vi "Actor Core.vi"(8 "error in":errorcluster, 11 "Panel Object Actions UI in":refnum<class "Panel Object Actions UI.lvclass">) -> (0 "error out":errorcluster, 3 "Actor out":refnum<class "Actor.lvclass">)   [LabVIEW 2015, in "Panel Object Actions UI.lvlib" / "Panel Object Actions UI.lvclass"]
doc: "The user interface for this panel.\n\n----\nPlease see the following web address for additional documentation and tutorial information:\nhttp://www.mooregoodideas.com/mgi-panel-manager/\n\nAuthor: Derek Trepanier\n\nCopyright (c) 2018, Moore Good Ideas, Inc.\n\nAll rights reserved.\n\nRedistribution and use in source and binary forms, with or without modification, are permitted provided that the following conditions are met:\n\n * Redistributions of source code must retain the above copyright notice, this list of conditions and the following disclaimer.\n * Redistributions in binary form must reproduce the above copyright notice, this list of conditions and the following disclaimer in the documentation and/or other materials provided with the distribution.\n * Neither the name of Moore Good Ideas, Inc. nor the names of its contributors may be used to endorse or promote products derived from this software without specific prior written permission.\n\nTHIS SOFTWARE IS PROVIDED BY THE COPYRIGHT HOLDERS AND CONTRIBUTORS \"AS IS\" AND ANY EXPRESS OR IMPLIED WARRANTIES, INCLUDING, BUT NOT LIMITED TO, THE IMPLIED WARRANTIES OF MERCHANTABILITY AND FITNESS FOR A PARTICULAR PURPOSE ARE DISCLAIMED. IN NO EVENT SHALL THE COPYRIGHT OWNER OR CONTRIBUTORS BE LIABLE FOR ANY DIRECT, INDIRECT, INCIDENTAL, SPECIAL, EXEMPLARY, OR CONSEQUENTIAL DAMAGES (INCLUDING, BUT NOT LIMITED TO, PROCUREMENT OF SUBSTITUTE GOODS OR SERVICES; LOSS OF USE, DATA, OR PROFITS; OR BUSINESS INTERRUPTION) HOWEVER CAUSED AND ON ANY THEORY OF LIABILITY, WHETHER IN CONTRACT, STRICT LIABILITY, OR TORT (INCLUDING NEGLIGENCE OR OTHERWISE) ARISING IN ANY WAY OUT OF THE USE OF THIS SOFTWARE, EVEN IF ADVISED OF THE POSSIBILITY OF SUCH DAMAGE."
uses:
  Panel Object Actions UI.lvclass
  <vilib>/ActorFramework/Actor/Actor.lvclass
  Classes/Panel Object/Panel Object.lvclass
  <vilib>/ActorFramework/Actor/Actor.lvclass/Actor.ctl
  Panel Object Actions UI.lvclass/Panel Object Actions UI.ctl
  <vilib>/ActorFramework/Message Enqueuer/Message Enqueuer.lvclass/Message Enqueuer.ctl
  Typedefs/Scrollbar Visibility--Enum.ctl
  Classes/Panel Object/Align Type--Enum.ctl
  Classes/Panel Object/Distribution Type--Enum.ctl
  <vilib>/ActorFramework/Message Enqueuer/Enqueue.vi
  <vilib>/ActorFramework/Message Priority Queue/Priority Enqueue.vi
  Pane Relief Main UI/Pane Relief Main UI Messages/Panel Object Settings Changed Msg/Panel Object Settings Changed Msg.lvclass
  <vilib>/MGI/Panel Manager/Panel Actor/Panel Actor/Panel Actor.lvclass
panel:
  in  "Scrollbars Off Runtime":bool
  in  "Scrollbars Off":bool
  in  "Unlock Splitters":bool
  in  "Lock Splitters":bool
  in  "Horizontal Gap":bool
  in  "Vertical Gap":bool
  in  "Scrollbars On":bool
  in  "Origin To (0,0)":bool
  in  "Align Right":bool
  in  "Align Bottom":bool
  in  "Align Left":bool
  in  "Align Top":bool
  in  "Color":u32(colorbox)
  # "Align & Distribute"
  # "Origin"
  # "Lock"
  # "Scrollbar"
  # "Color"
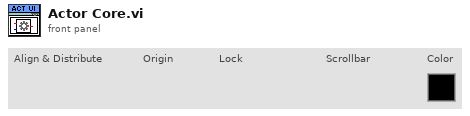
[diagram p1: front panel]
types:
  T1 = cluster{"Event Registration Refnum":refnum<event-registration>, "Pnl Actor":refnum<event-registration>}
  T2 = typedef "Scrollbar Visibility--Enum.ctl" = enum16{"On", "Off", "Off While Running"}
  T3 = typedef "Panel Object.lvclass/Align Type--Enum.ctl" = enum16{"Top", "Bottom", "Left", "Right"}
  T4 = typedef "Panel Object.lvclass/Distribution Type--Enum.ctl" = enum16{"Vertical", "Horizontal"}
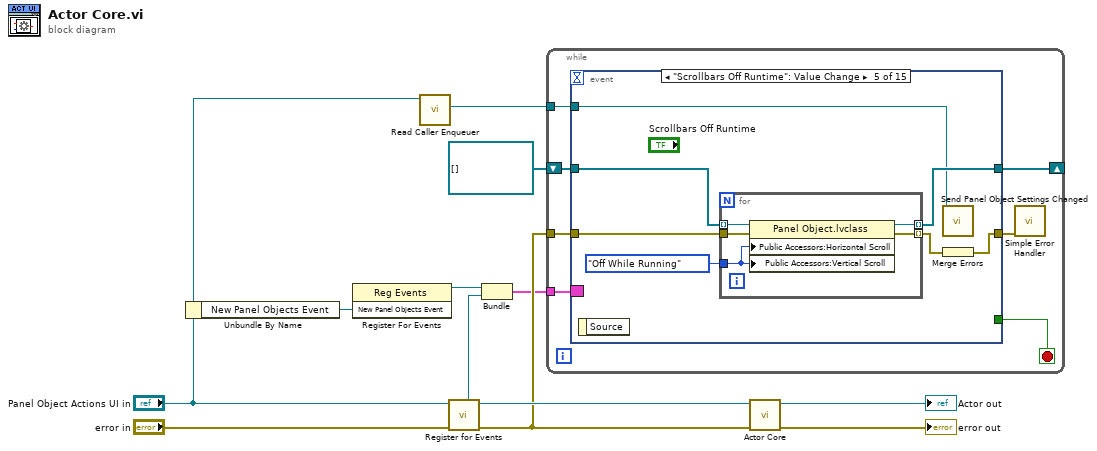
[diagram p0: block diagram]
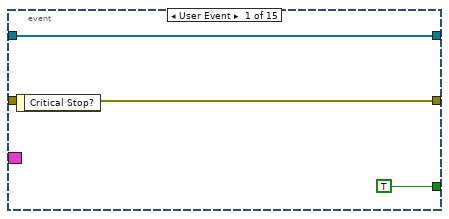
[diagram p2: hidden frame]
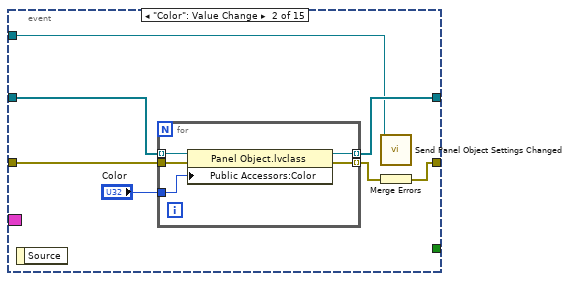
[diagram p3: hidden frame]
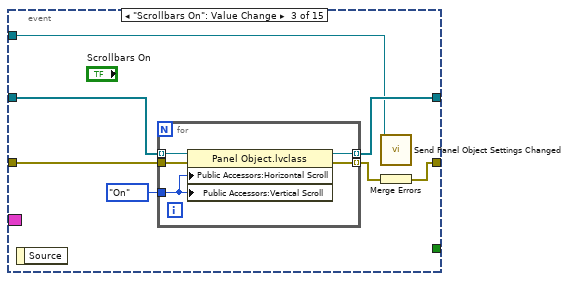
[diagram p4: hidden frame]
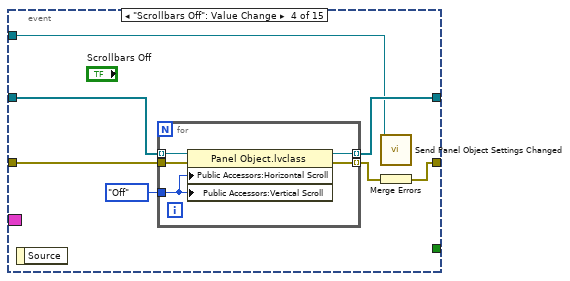
[diagram p5: hidden frame]
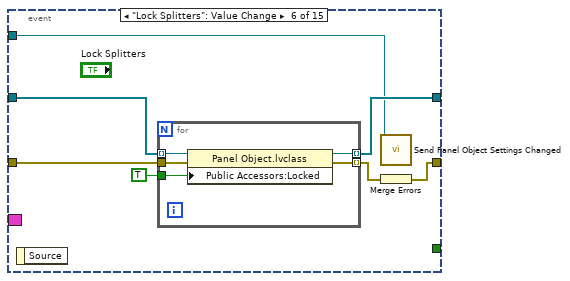
[diagram p6: hidden frame]
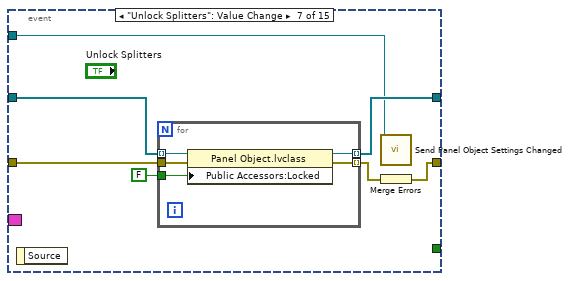
[diagram p7: hidden frame]
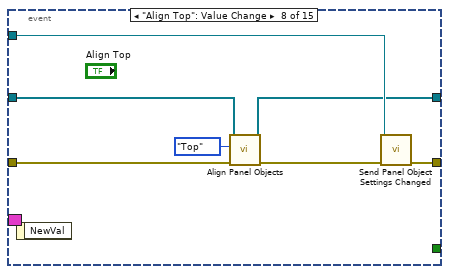
[diagram p8: hidden frame]
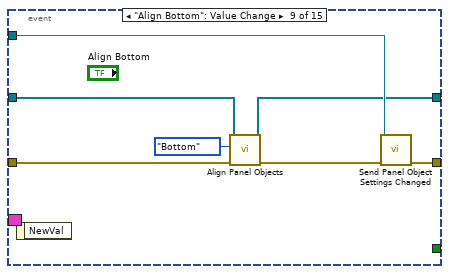
[diagram p9: hidden frame]
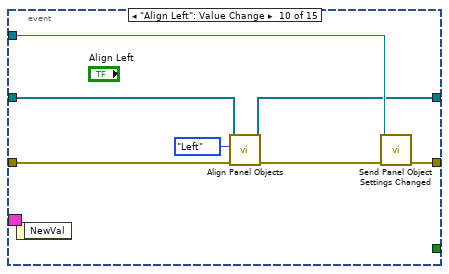
[diagram p10: hidden frame]
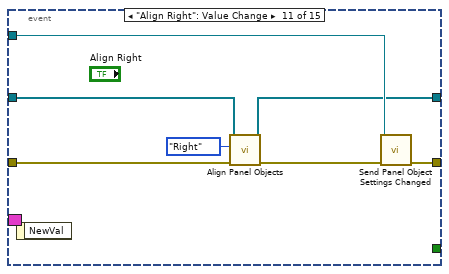
[diagram p11: hidden frame]
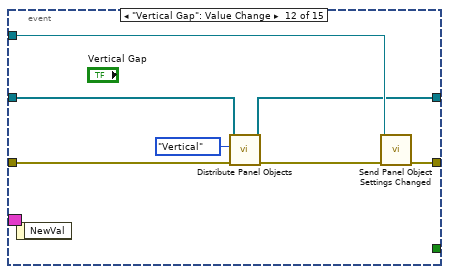
[diagram p12: hidden frame]
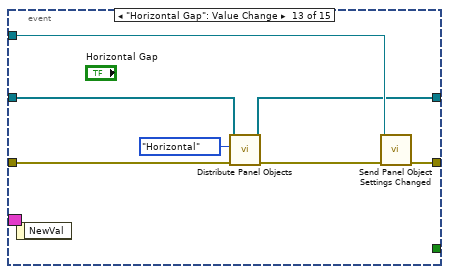
[diagram p13: hidden frame]
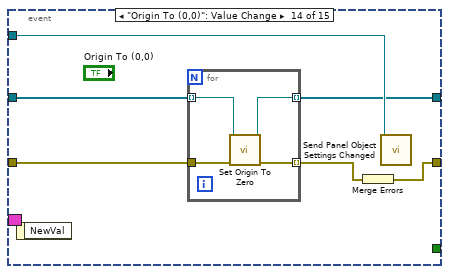
[diagram p14: hidden frame]
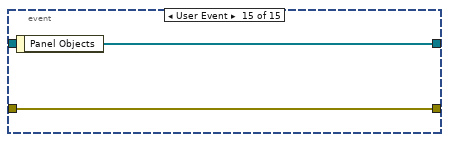
[diagram p15: hidden frame]
diagram:
  n1 = Unbundle By Name("Panel Object Actions UI in") -> ("New Panel Objects Event"=w6:refnum<user-event>)
  n2 = register-events(w6) -> (reference out=w10:refnum<event-registration>)  [unwired: 2 in, 1 out]
  n3 = call <vilib>:"Read Caller Enqueuer.vi"("Actor"="Panel Object Actions UI in") -> ("Caller Enqueuer"=w3:refnum<class "Message Enqueuer.lvclass">)  [unwired: 10 in]
  n4 = call <vilib>:"Register for Events.vi"("Error In"="error in", "Panel Actor in"="Panel Object Actions UI in") -> ("Error Out"=w5:errorcluster, "Panel Actor out"=w8:refnum<class "Panel Object Actions UI.lvclass">, "Pnl Actor"=w9:refnum<event-registration>)  [unwired: 6 in, 1 out]
  n5 = Bundle("Event Registration Refnum"=w10, "Pnl Actor"=w9) -> (w4:T1)  [unwired: 1 in]
  n6 = while {
    tunnel: w4 -> [w19]
    tunnel: w3 -> [w16]
    shift-right: [w15] -> _
    shift-left: refnum<class "Panel Object.lvclass">[] [] ("Panel Objects") -> [w14]
    tunnel: w5 -> [w17]
    stop <- w18 stop-if-true
    n7 = event shown="[4] \"Scrollbars Off Runtime\": Value Change" {
      selector: w19 -> [_ _ _ _ _ _ _ _ _ _ _ _ _ _ _]
      dyn-events: _ -> [_ _ _ _ _ _ _ _ _ _ _ _ _ _ _]
      timeout: _ -> [_ _ _ _ _ _ _ _ _ _ _ _ _ _ _]
      tunnel: [TRUE _ _ _ _ _ _ _ _ _ _ _ _ _ _] -> w18
      tunnel: w17 -> [w21 w28 w40 w52 w64 w76 w88 w99 w105 w111 w117 w123 w129 w135 w142]
      tunnel: [w21 w23 w35 w47 w59 w71 w83 w95 w101 w107 w113 w119 w125 w131 w142] -> w13
      tunnel: w16 -> [_ w26 w38 w50 w62 w74 w86 w100 w106 w112 w118 w124 w130 w136 _]
      tunnel: [w20 w27 w39 w51 w63 w75 w87 w97 w103 w109 w115 w121 w127 w133 w141] -> w15
      tunnel: w14 -> [w20 w29 w41 w53 w65 w77 w89 w98 w104 w110 w116 w122 w128 w134 _]
      event User Event {
        n8 = event-data() -> ()  [unwired: 1 in, 1 out]
      }
      event "Color": Value Change {
        n9 = event-data() -> ()  [unwired: 1 in, 1 out]
        n10 = for {
          tunnel: w29 -> [w34] mode=indexing
          tunnel: [w31] -> w27 mode=indexing
          tunnel: "Color" -> [w30]
          tunnel: w28 -> [w32]
          tunnel: [w33] -> w24 mode=indexing
          n11 = property class="Panel Object.lvclass"(reference=w34, error in=w32, "Public Accessors:Color"=w30) -> (reference out=w31:refnum<class "Panel Object.lvclass">, error out=w33:errorcluster)
        }
        n12 = call "Send Panel Object Settings Changed.vi"("Message Enqueuer"=w26) -> ()  [unwired: 9 in, 2 out]
        n13 = Merge Errors(w24) -> (w23:errorcluster)
      }
      event "Scrollbars On": Value Change {
        n14 = event-data() -> ()  [unwired: 1 in, 1 out]
        n15 = for {
          tunnel: w41 -> [w46] mode=indexing
          tunnel: [w43] -> w39 mode=indexing
          tunnel: Scrollbar_Visibility--Enum."On" ("Vertical Scroll") -> [w42]
          tunnel: w40 -> [w44]
          tunnel: [w45] -> w36 mode=indexing
          n16 = property class="Panel Object.lvclass"(reference=w46, error in=w44, "Public Accessors:Horizontal Scroll"=w42, "Public Accessors:Vertical Scroll"=w42) -> (reference out=w43:refnum<class "Panel Object.lvclass">, error out=w45:errorcluster)
        }
        n17 = call "Send Panel Object Settings Changed.vi"("Message Enqueuer"=w38) -> ()  [unwired: 9 in, 2 out]
        n18 = Merge Errors(w36) -> (w35:errorcluster)
      }
      event "Scrollbars Off": Value Change {
        n19 = event-data() -> ()  [unwired: 1 in, 1 out]
        n20 = for {
          tunnel: w53 -> [w58] mode=indexing
          tunnel: [w55] -> w51 mode=indexing
          tunnel: Scrollbar_Visibility--Enum."Off" ("Vertical Scroll") -> [w54]
          tunnel: w52 -> [w56]
          tunnel: [w57] -> w48 mode=indexing
          n21 = property class="Panel Object.lvclass"(reference=w58, error in=w56, "Public Accessors:Horizontal Scroll"=w54, "Public Accessors:Vertical Scroll"=w54) -> (reference out=w55:refnum<class "Panel Object.lvclass">, error out=w57:errorcluster)
        }
        n22 = call "Send Panel Object Settings Changed.vi"("Message Enqueuer"=w50) -> ()  [unwired: 9 in, 2 out]
        n23 = Merge Errors(w48) -> (w47:errorcluster)
      }
      event "Scrollbars Off Runtime": Value Change {
        n24 = event-data() -> ()  [unwired: 1 in, 1 out]
        n25 = for {
          tunnel: w65 -> [w70] mode=indexing
          tunnel: [w67] -> w63 mode=indexing
          tunnel: Scrollbar_Visibility--Enum."Off While Running" ("Vertical Scroll") -> [w66]
          tunnel: w64 -> [w68]
          tunnel: [w69] -> w60 mode=indexing
          n26 = property class="Panel Object.lvclass"(reference=w70, error in=w68, "Public Accessors:Horizontal Scroll"=w66, "Public Accessors:Vertical Scroll"=w66) -> (reference out=w67:refnum<class "Panel Object.lvclass">, error out=w69:errorcluster)
        }
        n27 = call "Send Panel Object Settings Changed.vi"("Message Enqueuer"=w62) -> ()  [unwired: 9 in, 2 out]
        n28 = Merge Errors(w60) -> (w59:errorcluster)
      }
      event "Lock Splitters": Value Change {
        n29 = event-data() -> ()  [unwired: 1 in, 1 out]
        n30 = for {
          tunnel: w77 -> [w82] mode=indexing
          tunnel: [w79] -> w75 mode=indexing
          tunnel: TRUE -> [w78]
          tunnel: w76 -> [w80]
          tunnel: [w81] -> w72 mode=indexing
          n31 = property class="Panel Object.lvclass"(reference=w82, error in=w80, "Public Accessors:Locked"=w78) -> (reference out=w79:refnum<class "Panel Object.lvclass">, error out=w81:errorcluster)
        }
        n32 = call "Send Panel Object Settings Changed.vi"("Message Enqueuer"=w74) -> ()  [unwired: 9 in, 2 out]
        n33 = Merge Errors(w72) -> (w71:errorcluster)
      }
      event "Unlock Splitters": Value Change {
        n34 = event-data() -> ()  [unwired: 1 in, 1 out]
        n35 = for {
          tunnel: w89 -> [w94] mode=indexing
          tunnel: [w91] -> w87 mode=indexing
          tunnel: FALSE -> [w90]
          tunnel: w88 -> [w92]
          tunnel: [w93] -> w84 mode=indexing
          n36 = property class="Panel Object.lvclass"(reference=w94, error in=w92, "Public Accessors:Locked"=w90) -> (reference out=w91:refnum<class "Panel Object.lvclass">, error out=w93:errorcluster)
        }
        n37 = call "Send Panel Object Settings Changed.vi"("Message Enqueuer"=w86) -> ()  [unwired: 9 in, 2 out]
        n38 = Merge Errors(w84) -> (w83:errorcluster)
      }
      event "Align Top": Value Change {
        n39 = event-data() -> ()  [unwired: 1 in, 1 out]
        n40 = call "Align Panel Objects.vi"("error in (no error)"=w99, "Align Type"=Align_Type--Enum."Top", "Panel Objects in"=w98) -> ("error out"=w95:errorcluster, "Panel Objects out"=w97:refnum<class "Panel Object.lvclass">[])  [unwired: 7 in]
        n41 = call "Send Panel Object Settings Changed.vi"("Message Enqueuer"=w100) -> ()  [unwired: 9 in, 2 out]
      }
      event "Align Bottom": Value Change {
        n42 = event-data() -> ()  [unwired: 1 in, 1 out]
        n43 = call "Align Panel Objects.vi"("error in (no error)"=w105, "Align Type"=Align_Type--Enum."Bottom", "Panel Objects in"=w104) -> ("error out"=w101:errorcluster, "Panel Objects out"=w103:refnum<class "Panel Object.lvclass">[])  [unwired: 7 in]
        n44 = call "Send Panel Object Settings Changed.vi"("Message Enqueuer"=w106) -> ()  [unwired: 9 in, 2 out]
      }
      event "Align Left": Value Change {
        n45 = event-data() -> ()  [unwired: 1 in, 1 out]
        n46 = call "Align Panel Objects.vi"("error in (no error)"=w111, "Align Type"=Align_Type--Enum."Left", "Panel Objects in"=w110) -> ("error out"=w107:errorcluster, "Panel Objects out"=w109:refnum<class "Panel Object.lvclass">[])  [unwired: 7 in]
        n47 = call "Send Panel Object Settings Changed.vi"("Message Enqueuer"=w112) -> ()  [unwired: 9 in, 2 out]
      }
      event "Align Right": Value Change {
        n48 = event-data() -> ()  [unwired: 1 in, 1 out]
        n49 = call "Align Panel Objects.vi"("error in (no error)"=w117, "Align Type"=Align_Type--Enum."Right", "Panel Objects in"=w116) -> ("error out"=w113:errorcluster, "Panel Objects out"=w115:refnum<class "Panel Object.lvclass">[])  [unwired: 7 in]
        n50 = call "Send Panel Object Settings Changed.vi"("Message Enqueuer"=w118) -> ()  [unwired: 9 in, 2 out]
      }
      event "Vertical Gap": Value Change {
        n51 = event-data() -> ()  [unwired: 1 in, 1 out]
        n52 = call "Distribute Panel Objects.vi"("error in (no error)"=w123, "Distribution Type"=Distribution_Type--Enum."Vertical", "Panel Objects in"=w122) -> ("error out"=w119:errorcluster, "Panel Objects out"=w121:refnum<class "Panel Object.lvclass">[])  [unwired: 7 in]
        n53 = call "Send Panel Object Settings Changed.vi"("Message Enqueuer"=w124) -> ()  [unwired: 9 in, 2 out]
      }
      event "Horizontal Gap": Value Change {
        n54 = event-data() -> ()  [unwired: 1 in, 1 out]
        n55 = call "Distribute Panel Objects.vi"("error in (no error)"=w129, "Distribution Type"=Distribution_Type--Enum."Horizontal", "Panel Objects in"=w128) -> ("error out"=w125:errorcluster, "Panel Objects out"=w127:refnum<class "Panel Object.lvclass">[])  [unwired: 7 in]
        n56 = call "Send Panel Object Settings Changed.vi"("Message Enqueuer"=w130) -> ()  [unwired: 9 in, 2 out]
      }
      event "Origin To (0,0)": Value Change {
        n57 = event-data() -> ()  [unwired: 1 in, 1 out]
        n58 = for {
          tunnel: w134 -> [w138] mode=indexing
          tunnel: [w137] -> w133 mode=indexing
          tunnel: w135 -> [w140]
          tunnel: [w139] -> w132 mode=indexing
          n59 = call-dynamic "Set Origin To Zero.vi"("error in (no error)"=w140, "Panel Object in"=w138) -> ("error out"=w139:errorcluster, "Panel Object out"=w137:refnum<class "Panel Object.lvclass">)  [unwired: 8 in]
        }
        n60 = Merge Errors(w132) -> (w131:errorcluster)
        n61 = call "Send Panel Object Settings Changed.vi"("Message Enqueuer"=w136) -> ()  [unwired: 9 in, 2 out]
      }
      event User Event {
        n62 = event-data() -> ("Panel Objects"=w141:refnum<class "Panel Object.lvclass">[])  [unwired: 1 in]
      }
    }
    n63 = call <vilib>:"Simple Error Handler.vi"("error in (no error)"=w13) -> ()  [unwired: 4 in, 5 out]
  }
  n64 = call-parent "Actor Core.vi"("error in"=w5, "Panel Actor in"=w8) -> ("error out"=→"error out":errorcluster, "Actor out"=→"Actor out":refnum<class "Actor.lvclass">)  [unwired: 8 in]
